vi "DNS-SD mDNS Query.vi"(7 "timeout, ms (5000)":i32=5000, 8 "error in (no error)":errorcluster, 9 "instance name (any)":string, 10 "max number of instances (all)":u32, 11 "service.domain":string="_http._tcp.local") -> (0 "error out":errorcluster)   [LabVIEW 2015, in "PL DNS Client.lvlib"]
doc: "Discovers <b>service instances</b> specified by <b>service.domain</b>. <b>max number of instances</b> and <b>instance name</b> and can be used to limit returned service instances by number and occurense of specific string in instance name."
uses:
  PL DNS Client.lvlib
panel:
  out "service instances":T1(array[cluster])
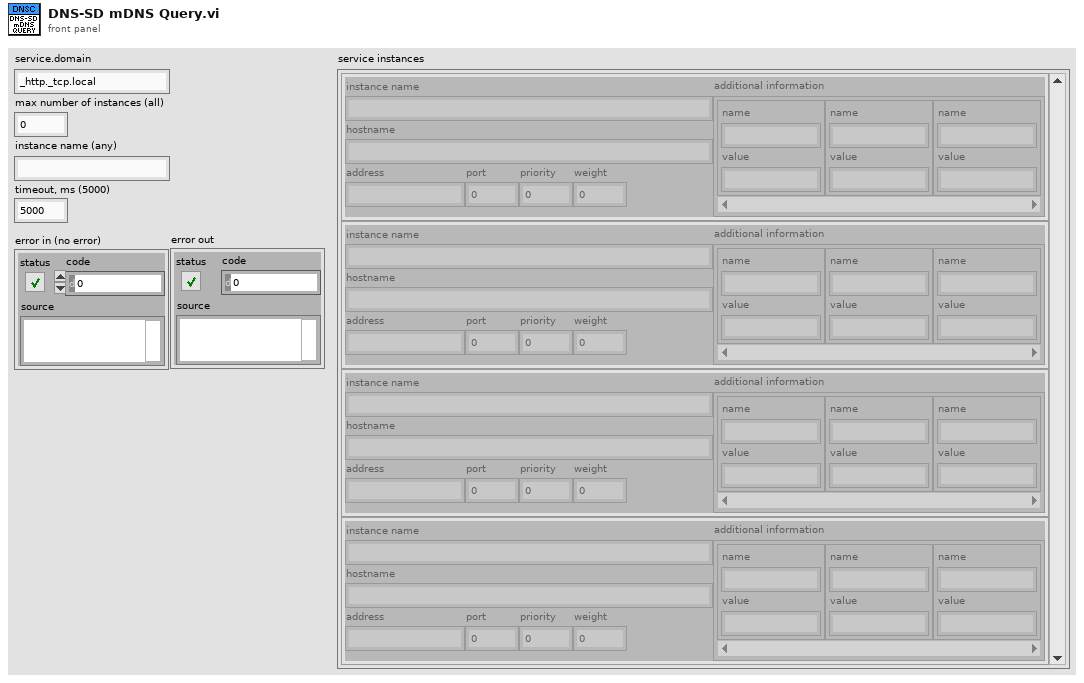
[diagram p1: front panel]
types:
  T1 = cluster{"instance name":string, "hostname":string, "address":string, "port":u16, "priority":u16, "weight":u16, "additional information":cluster{"name":string, "value":string}[]}[]
  T2 = cluster{"service.domain":string, "type":u16, "class":u16}
  T3 = cluster{"service.domain":string, "type":u16, "class":u16}[]
  T4 = cluster{"header":cluster{"opcode":u8, "recursion desired":bool}, cluster{"service.domain":string, "type":u16, "class":u16}[]}
  T5 = cluster{"instance name":string, "hostname":string, "address":string, "port":u16, "priority":u16, "weight":u16, "additional information":cluster{"name":string, "value":string}[]}
  T6 = cluster{"message":string, "header":cluster{"id":u16, "response":bool, "opcode":u8, "authoritative answer":bool, "truncation":bool, "recursion desired":bool, "recursion available":bool, "response code":u16}, "answers":cluster{"name":string, "type":u16, "class":u16, "ttl":u32, "data length":u16, "data offset":u16}[], "authority records":cluster{"name":string, "type":u16, "class":u16, "ttl":u32, "data length":u16, "data offset":u16}[], "additional records":cluster{"name":string, "type":u16, "class":u16, "ttl":u32, "data length":u16, "data offset":u16}[]}
  T7 = cluster{"hostname":string, "type":u16, "class":u16}
  T8 = cluster{"hostname":string, "type":u16, "class":u16}[]
  T9 = cluster{"header":cluster{"opcode":u8, "recursion desired":bool}, cluster{"hostname":string, "type":u16, "class":u16}[]}
  T10 = cluster{"message":string, "header":cluster{"id":u16, "response":bool, "opcode":u8, "authoritative answer":bool, "truncation":bool, "recursion desired":bool, "recursion available":bool, "response code":u16}, "answers":cluster{"name":string, "type":u16, "class":u16, "ttl":u32, "data length":u16, "data offset":u16}[], "authority records":cluster{"name":string, "type":u16, "class":u16, "ttl":u32, "data length":u16, "data offset":u16}[], "additional records":cluster{"name":string, "type":u16, "class":u16, "ttl":u32, "data length":u16, "data offset":u16}[]}[]
  T11 = cluster{"name":string, "type":u16, "class":u16, "ttl":u32, "data length":u16, "data offset":u16}[]
  T12 = cluster{"name":string, "type":u16, "class":u16, "ttl":u32, "data length":u16, "data offset":u16}
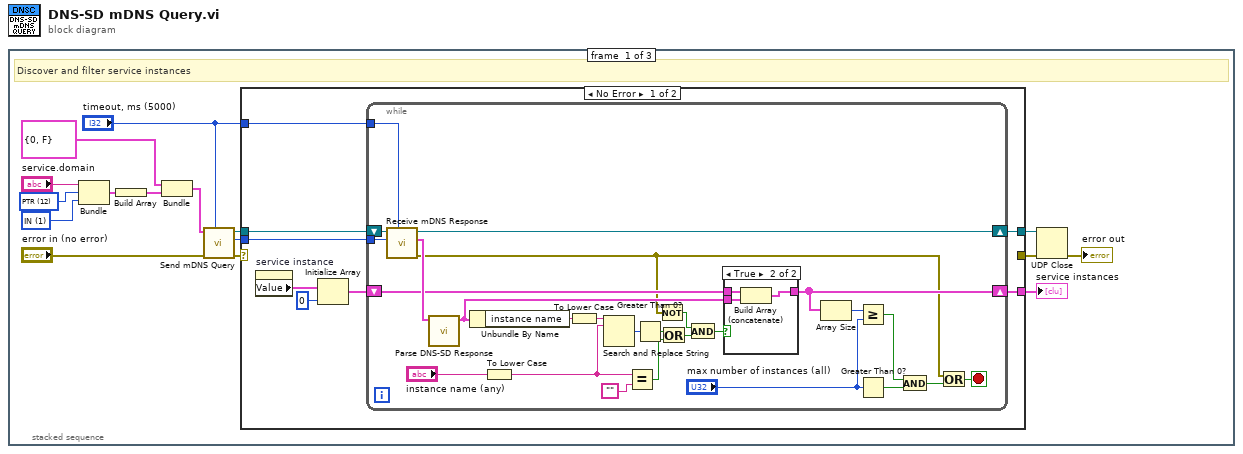
[diagram p0: block diagram]
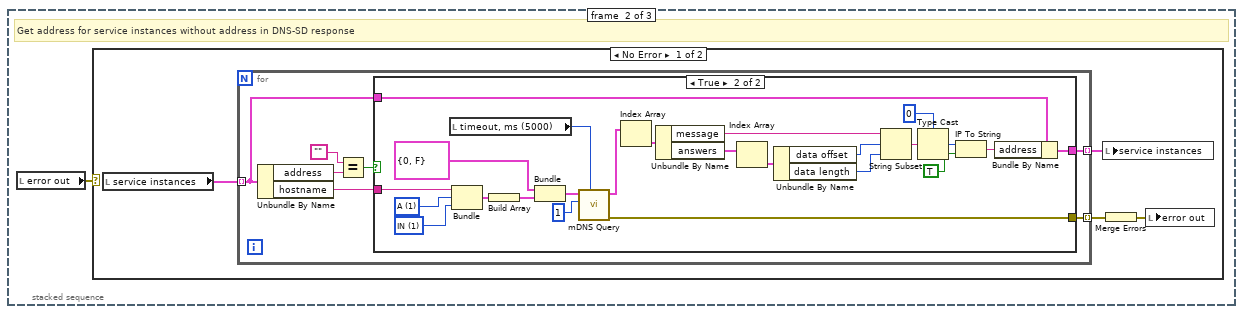
[diagram p4: hidden frame]
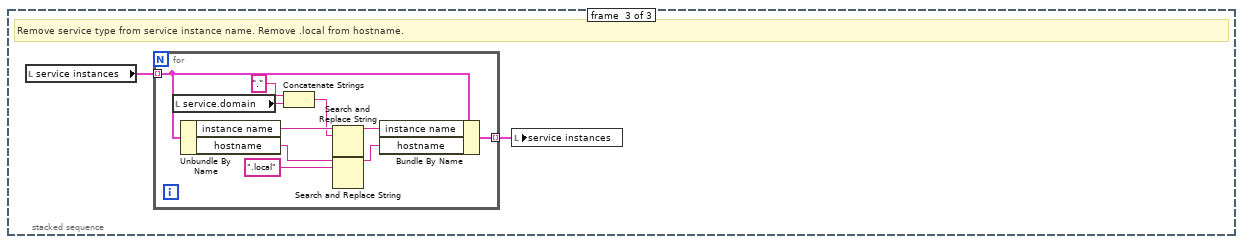
[diagram p7: hidden frame]
diagram:
  n1 = stacked-sequence {
    frame #0 {
      w14 = u16 12 items=["A"=1, "NS"=2, "MD"=3, "MF"=4, "CNAME"=5, "SOA"=6, "MB"=7, "MG"=8, "MR"=9, "NULL"=10, "WKS"=11, "PTR"=12, "HINFO"=13, "MINFO"=14, "MX"=15, "TXT"=16, "RP"=17, "AFSDB"=18, "X25"=19, "ISDN"=20, "RT"=21, "NSAP"=22, "NSAP-PTR"=23, "SIG"=24, "KEY"=25, "PX"=26, "GPOS"=27, "AAAA"=28, "LOC"=29, "NXT"=30, "EID"=31, "NIMLOC"=32, "SRV"=33, "ATMA"=34, "NAPTR"=35, "KX"=36, "CERT"=37, "A6"=38, "DNAME"=39, "SINK"=40, "OPT"=41, "APL"=42, "DS"=43, "SSHFP"=44, "IPSECKEY"=45, "RRSIG"=46, "NSEC"=47, "DNSKEY"=48, "DHCID"=49, "NSEC3"=50, "NSEC3PARAM"=51, "TLSA"=52, "SMIMEA"=53, "HIP"=55, "NINFO"=56, "RKEY"=57, "TALINK"=58, "CDS"=59, "CDNSKEY"=60, "OPENPGPKEY"=61, "CSYNC"=62, "ZONEMD"=63, "SVCB"=64, "HTTPS"=65, "SPF"=99, "UINFO"=100, "UID"=101, "GID"=102, "UNSPEC"=103, "NID"=104, "L32"=105, "L64"=106, "LP"=107, "EUI48"=108, "EUI64"=109, "TKEY"=249, "TSIG"=250, "IXFR"=251, "AXFR"=252, "MAILB"=253, "MAILA"=254, "*"=255, "URI"=256, "CAA"=257, "AVC"=258, "DOA"=259, "AMTRELAY"=260, "TA"=32768, "DLV"=32769] ("type")
      w13 = u16 1 items=["IN"=1, "CH"=3, "HS"=4, "NONE"=254, "*"=255] ("class")
      # "Discover and filter service instances"
      n2 = Bundle("service.domain"="service.domain", "type"=w14, "class"=w13) -> (w12:T2)  [unwired: 1 in]
      n3 = Build Array(w12) -> (w11:T3)
      n4 = Bundle("header"=cluster{"opcode":u8, "recursion desired":bool} {"opcode"=0, "recursion desired"=FALSE}, w11) -> (w10:T4)  [unwired: 1 in]
      n5 = call "Send mDNS Query.vi"("timeout, ms (5000)"="timeout, ms (5000)", "error in (no error)"="error in (no error)", "query"=w10) -> ("error out"=w8:errorcluster, "query id"=w6:u16, "connection ID"=w7:refnum<k16>)  [unwired: 6 in]
      n6 = case shown="No Error" w8 {
        selector: w8 -> [_ w55]
        tunnel: w7 -> [w24 w56]
        tunnel: w6 -> [w23 _]
        tunnel: [w22 w56] -> w5
        tunnel: [_ w55] -> w4
        tunnel: [w18 _] -> w2
        tunnel: "timeout, ms (5000)" -> [w17 _]
        frame No Error {
          n7 = property on="service instance" class="Clust (strict)"() -> ("Value"=w21:T5)  [unwired: 2 in, 2 out]
          n8 = Initialize Array(w21, 0 ("dimension size")) -> (w19:T1)
          n9 = while {
            shift-right: [w49] -> w22
            shift-left: w24 -> [w50]
            tunnel: w23 -> [w28]
            shift-right: [w37] -> w18
            shift-left: w19 -> [w40]
            tunnel: w17 -> [w27]
            stop <- w29 stop-if-true
            n10 = call "Receive mDNS Response.vi"("timeout, ms (5000)"=w27, "query id"=w28, "connection ID"=w50) -> ("error out"=w30:errorcluster, "response"=w48:T6, "connection ID out"=w49:refnum<k16>)  [unwired: 6 in]
            n11 = call "Parse DNS-SD Response.vi"("response"=w48) -> ("service instance"=w39:T5)  [unwired: 10 in]
            n12 = Unbundle By Name(w39) -> ("instance name"=w47:string)
            n13 = To Lower Case(string="instance name (any)") -> (all lower case string=w26:string)
            n14 = To Lower Case(string=w47) -> (all lower case string=w25:string)
            n15 = Search and Replace String(input string=w25, search string=w26) -> (number of replacements=w46:i32)  [unwired: 6 in, 3 out]
            n16 = Equal?(x=w26, y="") -> (x = y?=w42:bool)
            n17 = Greater Than 0?(x=w46) -> (x > 0?=w43:bool)
            n18 = Not(x=w30) -> (.not. x?=w32:bool)
            n19 = Or(x=w43, y=w42) -> (x .or. y?=w41:bool)
            n20 = And(x=w32, y=w41) -> (x .and. y?=w38:bool)
            n21 = case shown="True" w38 {
              tunnel: w40 -> [w51 w54]
              tunnel: [w51 w53] -> w37
              tunnel: w39 -> [_ w52]
              frame False {
              }
              frame True {
                n22 = Build Array (concatenate)(w54, w52) -> (w53:T1)
              }
            }
            n23 = Array Size(array=w37) -> (size(s)=w36:i32)
            n24 = Greater Or Equal?(x=w36, y="max number of instances (all)") -> (x >= y?=w35:bool)
            n25 = Greater Than 0?(x="max number of instances (all)") -> (x > 0?=w33:bool)
            n26 = And(x=w35, y=w33) -> (x .and. y?=w31:bool)
            n27 = Or(x=w30, y=w31) -> (x .or. y?=w29:bool)
          }
        }
        frame Error {
        }
      }
      "service instances" <- w2
      n28 = UDP Close(connection ID=w5, 8:w4) -> (error out=→"error out":errorcluster)  [unwired: 1 out]
    }
    frame #1 {
      # "Get address for service instances without address in DNS-SD response"
      n29 = local read "error out"() -> (w57:errorcluster)
      n30 = case shown="No Error" w57 {
        frame No Error {
          n31 = local read "service instances"() -> (w61:T1)
          n32 = for {
            tunnel: w61 -> [w66] mode=indexing
            tunnel: [w67] -> w60 mode=indexing
            tunnel: [w65] -> w58 mode=indexing
            n33 = Unbundle By Name(w66) -> ("address"=w64:string, "hostname"=w68:string)
            n34 = Equal?(x="", y=w64) -> (x = y?=w63:bool)
            n35 = case shown="True" w63 {
              tunnel: w68 -> [_ w87]
              tunnel: [_ w85] -> w67
              tunnel: w66 -> [w69 w84]
              tunnel: [w69 w71] -> w65
              frame False {
              }
              frame True {
                w92 = u16 1 items=["A"=1, "NS"=2, "MD"=3, "MF"=4, "CNAME"=5, "SOA"=6, "MB"=7, "MG"=8, "MR"=9, "NULL"=10, "WKS"=11, "PTR"=12, "HINFO"=13, "MINFO"=14, "MX"=15, "TXT"=16, "RP"=17, "AFSDB"=18, "X25"=19, "ISDN"=20, "RT"=21, "NSAP"=22, "NSAP-PTR"=23, "SIG"=24, "KEY"=25, "PX"=26, "GPOS"=27, "AAAA"=28, "LOC"=29, "NXT"=30, "EID"=31, "NIMLOC"=32, "SRV"=33, "ATMA"=34, "NAPTR"=35, "KX"=36, "CERT"=37, "A6"=38, "DNAME"=39, "SINK"=40, "OPT"=41, "APL"=42, "DS"=43, "SSHFP"=44, "IPSECKEY"=45, "RRSIG"=46, "NSEC"=47, "DNSKEY"=48, "DHCID"=49, "NSEC3"=50, "NSEC3PARAM"=51, "TLSA"=52, "SMIMEA"=53, "HIP"=55, "NINFO"=56, "RKEY"=57, "TALINK"=58, "CDS"=59, "CDNSKEY"=60, "OPENPGPKEY"=61, "CSYNC"=62, "ZONEMD"=63, "SVCB"=64, "HTTPS"=65, "SPF"=99, "UINFO"=100, "UID"=101, "GID"=102, "UNSPEC"=103, "NID"=104, "L32"=105, "L64"=106, "LP"=107, "EUI48"=108, "EUI64"=109, "TKEY"=249, "TSIG"=250, "IXFR"=251, "AXFR"=252, "MAILB"=253, "MAILA"=254, "*"=255, "URI"=256, "CAA"=257, "AVC"=258, "DOA"=259, "AMTRELAY"=260, "TA"=32768, "DLV"=32769] ("type")
                w91 = u16 1 items=["IN"=1, "CH"=3, "HS"=4, "NONE"=254, "*"=255] ("class")
                n36 = local read "timeout, ms (5000)"() -> (w86:i32)
                n37 = Bundle("hostname"=w87, "type"=w92, "class"=w91) -> (w90:T7)  [unwired: 1 in]
                n38 = Build Array(w90) -> (w89:T8)
                n39 = Bundle("header"=cluster{"opcode":u8, "recursion desired":bool} {"opcode"=0, "recursion desired"=FALSE}, w89) -> (w88:T9)  [unwired: 1 in]
                n40 = call "mDNS Query.vi"("timeout, ms (5000)"=w86, "max number of responses (all)"=u32 1, "request"=w88) -> ("error out"=w85:errorcluster, "responses"=w82:T10)  [unwired: 7 in]
                n41 = Index Array(array=w82) -> (element=w83:T6)  [unwired: 1 in]
                n42 = Unbundle By Name(w83) -> ("message"=w75:string, "answers"=w81:T11)
                n43 = Index Array(array=w81) -> (element=w80:T12)  [unwired: 1 in]
                n44 = Unbundle By Name(w80) -> ("data offset"=w74:u16, "data length"=w73:u16)
                n45 = String Subset(string=w75, offset (0)=w74, length (rest)=w73) -> (substring=w77:string)
                n46 = Type Cast(type=u32 0 ("net address"), x=w77) -> (*(type *) &x=w79:u32)
                n47 = IP To String(1:TRUE ("dot notation? (F)"), 2:w79) -> (0:w72:string)
                n48 = Bundle By Name(cluster=w84, "address"=w72) -> (w71:T5)
              }
            }
          }
          n49 = local write "service instances"(w58) -> ()
          n50 = Merge Errors(w60) -> (w59:errorcluster)
          n51 = local write "error out"(w59) -> ()
        }
        frame Error {
        }
      }
    }
    frame #2 {
      # "Remove service type from service instance name. Remove .local from hostname."
      n52 = local read "service instances"() -> (w95:T1)
      n53 = for {
        tunnel: w95 -> [w102] mode=indexing
        tunnel: [w99] -> w94 mode=indexing
        n54 = local read "service.domain"() -> (w104:string)
        n55 = Unbundle By Name(w102) -> ("instance name"=w105:string, "hostname"=w98:string)
        n56 = Concatenate Strings("." ("string"), w104) -> (w100:string)
        n57 = Search and Replace String(input string=w105, search string=w100) -> (result string=w101:string)  [unwired: 6 in, 3 out]
        n58 = Search and Replace String(input string=w98, search string=".local") -> (result string=w96:string)  [unwired: 6 in, 3 out]
        n59 = Bundle By Name(cluster=w102, "instance name"=w101, "hostname"=w96) -> (w99:T5)
      }
      n60 = local write "service instances"(w94) -> ()
    }
  }
